vi "Write Configuration from Variant Array.vi"(8 "error in":errorcluster, 10 "Configuration Variant Array":variant[](array[variant]), 11 "Master Controller in":refnum<class "EMS User Interface.lvclass">) -> (0 "error out":errorcluster, 3 "Master Controller out":refnum<class "EMS User Interface.lvclass">)   [LabVIEW 2018, in "EMS Generic Actor.lvlib" / "EMS Generic.lvclass"]
uses:
  EMS Generic.lvclass
  EMS User Interface Actor/EMS User Interface/EMS User Interface.lvclass
  C:/Program Files (x86)/National Instruments/LabVIEW 2018/vi.lib/ActorFramework/Actor/Actor.lvclass
  <vilib>/ORNL/CSEISMIC DDS/CSEISMIC DDS Base/Data Types/Controls/DeviceID.ctl
  <vilib>/ActorFramework/Actor/Actor.lvclass/Actor.ctl
  <vilib>/ActorFramework/Message Enqueuer/Message Enqueuer.lvclass/Message Enqueuer.ctl
  EMS User Interface Actor/EMS User Interface Messages/Write Nominal Frequency Msg/Write Nominal Frequency Msg.lvclass/Write Nominal Frequency Msg.ctl
  EMS User Interface Actor/EMS User Interface Messages/Write Nominal Voltage Msg/Write Nominal Voltage Msg.lvclass/Write Nominal Voltage Msg.ctl
  Dialog Actors/Devices to Load Actor/Devices to Load Messages/Return Devices to Load IDs Msg/Return Devices to Load IDs Msg.lvclass/Return Devices to Load IDs Msg.ctl
  EMS User Interface Actor/EMS User Interface Messages/Write VF Device ID Msg/Write VF Device ID Msg.lvclass/Write VF Device ID Msg.ctl
  <vilib>/ActorFramework/Message Enqueuer/Init from Existing Queue.vi
  <vilib>/ActorFramework/Message Enqueuer/Enqueue.vi
  Dialog Actors/Devices to Load Actor/Devices to Load Messages/Return Devices to Load IDs Msg/Send Return Devices to Load IDs.vi
  EMS User Interface Actor/EMS User Interface Messages/Write Nominal Frequency Msg/Write Nominal Frequency Msg.lvclass
  C:/Program Files (x86)/National Instruments/LabVIEW 2018/vi.lib/ActorFramework/Message/Message.lvclass
  EMS User Interface Actor/EMS User Interface Messages/Write Nominal Voltage Msg/Write Nominal Voltage Msg.lvclass
  EMS User Interface Actor/EMS User Interface Messages/Write Device IDs Msg/Write Device IDs Msg.lvclass
  C:/Users/Administrator/Desktop/2018LabVIEW EMS/Dialog Actors/Devices to Load Actor/Devices to Load Messages/Return Devices to Load IDs Msg/Return Devices to Load IDs Msg.lvclass
  Dialog Actors/Devices to Load Actor/Devices to Load Messages/Return Devices to Load IDs Msg/Return Devices to Load IDs Msg.lvclass
  EMS User Interface Actor/EMS User Interface Messages/Write VF Device ID Msg/Write VF Device ID Msg.lvclass
  <vilib>/ActorFramework/Message Priority Queue/Priority Enqueue.vi
  <vilib>/ActorFramework/Message Enqueuer/Message Enqueuer.lvclass
  <vilib>/ORNL/CSEISMIC DDS/CSEISMIC DDS Base/CSEISMIC DDS.lvclass
  <vilib>/ActorFramework/Actor/Actor.lvclass
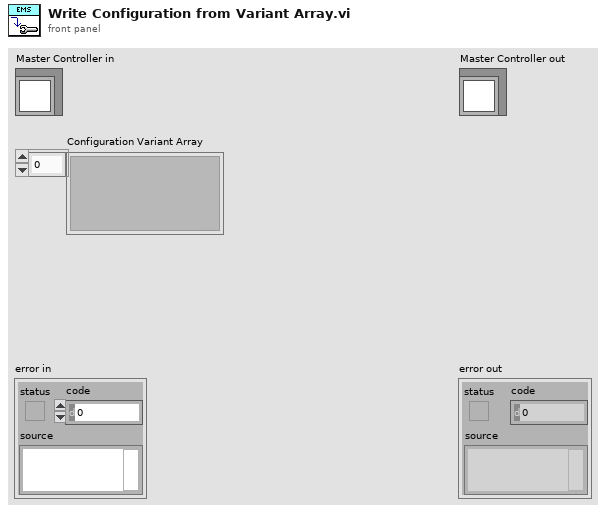
[diagram p1: front panel]
types:
  T1 = typedef "CSEISMIC DDS.lvlib/CSEISMIC DDS.lvclass/DeviceID.ctl" = string
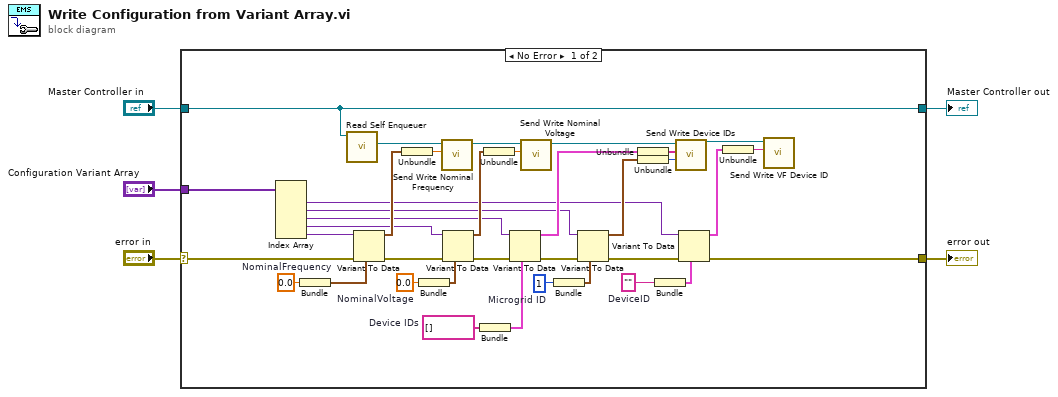
[diagram p0: block diagram]
diagram:
  n1 = case shown="No Error" "error in" {
    selector: "error in" -> [w14 w44]
    tunnel: [w10 w44] -> w4
    tunnel: [w16 w43] -> w2
    tunnel: "Master Controller in" -> [w16 w43]
    tunnel: "Configuration Variant Array" -> [w15 _]
    frame No Error {
      w8 = T1 ""  # DeviceID
      w34 = 0.0  # NominalFrequency
      w33 = 0.0  # NominalVoltage
      w25 = u8 1  # Microgrid ID
      w22 = T1[] []  # Device IDs
      n2 = Index Array(array=w15) -> (element #1=w9:variant, element #2=w17:variant, element #3=w19:variant, element #4=w31:variant, element #5=w30:variant)  [unwired: 5 in]
      n3 = Bundle("NominalFrequency"=w34) -> (w35:cluster{"NominalFrequency":dbl})  [unwired: 1 in]
      n4 = call <vilib>:"Read Self Enqueuer.vi"("Actor"=w16) -> ("Self Enqueuer"=w38:refnum<class "Message Enqueuer.lvclass">)  [unwired: 10 in]
      n5 = Variant To Data(error in=w14, type=w35, Variant=w30) -> (data=w36:cluster{"NominalFrequency":dbl}, error out=w29:errorcluster)
      n6 = Unbundle(w36) -> ("NominalFrequency"=w37:dbl)
      n7 = Bundle("NominalVoltage"=w33) -> (w32:cluster{"NominalVoltage":dbl})  [unwired: 1 in]
      n8 = call "Send Write Nominal Frequency.vi"("Nominal Frequency"=w37, "Message Enqueuer"=w38) -> ("Message Enqueuer out"=w39:refnum<class "Message Enqueuer.lvclass">)  [unwired: 8 in, 1 out]
      n9 = Variant To Data(error in=w29, type=w32, Variant=w31) -> (data=w40:cluster{"NominalVoltage":dbl}, error out=w28:errorcluster)
      n10 = Bundle("Device IDs"=w22) -> (w24:cluster{"Device IDs":T1[]})  [unwired: 1 in]
      n11 = Unbundle(w40) -> ("NominalVoltage"=w41:dbl)
      n12 = Variant To Data(error in=w28, type=w24, Variant=w19) -> (data=w21:cluster{"Device IDs":T1[]}, error out=w18:errorcluster)
      n13 = call "Send Write Nominal Voltage.vi"("Nominal Voltage"=w41, "Message Enqueuer"=w39) -> ("Message Enqueuer out"=w42:refnum<class "Message Enqueuer.lvclass">)  [unwired: 8 in, 1 out]
      n14 = Bundle("Microgrid ID"=w25) -> (w26:cluster{"Microgrid ID":u8})  [unwired: 1 in]
      n15 = Variant To Data(error in=w18, type=w26, Variant=w17) -> (data=w20:cluster{"Microgrid ID":u8}, error out=w11:errorcluster)
      n16 = Unbundle(w21) -> ("Device IDs"=w23:T1[])
      n17 = Unbundle(w20) -> ("Microgrid ID"=w27:u8)
      n18 = Bundle("DeviceID"=w8) -> (w12:cluster{"DeviceID":T1})  [unwired: 1 in]
      n19 = call "Send Write Device IDs.vi"("Microgrid ID"=w27, "Device IDs"=w23, "Message Enqueuer"=w42) -> ("Message Enqueuer out"=w13:refnum<class "Message Enqueuer.lvclass">)  [unwired: 7 in, 1 out]
      n20 = Variant To Data(error in=w11, type=w12, Variant=w9) -> (data=w7:cluster{"DeviceID":T1}, error out=w10:errorcluster)
      n21 = Unbundle(w7) -> ("DeviceID"=w6:T1)
      n22 = call "Send Write VF Device ID.vi"("VF Device ID"=w6, "Message Enqueuer"=w13) -> ()  [unwired: 8 in, 2 out]
    }
    frame Error {
    }
  }
  "error out" <- w4
  "Master Controller out" <- w2
